vi "Load and Vin SMU Measurement T16.vi"() -> ()   [LabVIEW 2021, in "Dep T16.lvlib"]
doc: "Demonstrates how to use the DC Voltage Output Function to force an output voltage. This example initializes a session, configures the Output Function, Sense, Autorange, Voltage Level and Current Limit, initiates generation, waits for a specified delay, and measures the voltage and current output. This example uses Single Point source mode."
uses:
  Dep T16.lvlib
  controls/Temp T16.ctl
  DMM/DMM T16.lvlib
panel:
  in  "Tektronix Scope":refnum<visa-resource-name>
  out "Division Number":i32
  in  "Sample Rate":dbl=3125000000.0
  in  "Maximum Record Length":dbl=250000000.0 format="%#_6e"
  out "SMU Measurement":dbl format="%.6p"
  in  "SMU DMM":refnum<k15>="Dev1"
  in  "SMU DMM Measurement":T1(ring)
  in  "SMU Resolution in Digits":dbl(ring)=5.5 items=["3 1/2"=3.5, "4 1/2"=4.5, "5 1/2"=5.5, "6 1/2"=6.5, "7 1/2"=7.5]
  out "Load Voltage":dbl caption="SMU Measurement" format="%.6p"
  in  "Load DMM":refnum<k15>="Dev1"
  in  "Load DMM Measurement":T1(ring) caption="SMU DMM Measurement"
  in  "Load SMU":refnum<k15>="Dev1"
  in  "Load SMU Channel":string="0"
  out "Load SMU Current":dbl
  out "Load SMU Voltage":dbl
  in  "error in":errorcluster
  out "error out":errorcluster
  out "Voltage Measurement":dbl caption="Vin SMU Voltage"
  out "Current Measurement":dbl caption="Vin SMU Current"
  in  "Current Limit":dbl=0.01 format="%.3p"
  in  "Voltage Level":dbl=2.0 format="%.5p"
  in  "Vin SMU Channel":string="0"
  in  "Vin SMU":refnum<k15>="Dev1"
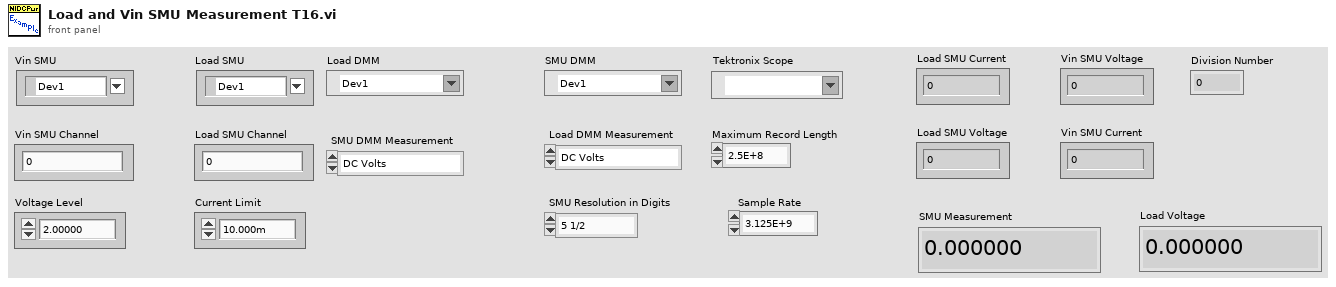
[diagram p1: front panel]
types:
  T1 = enum16{"DC Volts", "AC Volts", "DC Current", "AC Current", "2-wire Resistance", "4-wire Resistance", "Diode", "Frequency", "Period", "AC Volts DC Coupled", "Capacitance", "Inductance", "Temperature"}
  T2 = typedef "Temp T16.ctl" = cluster{"Read?":bool, "Temp":i32}
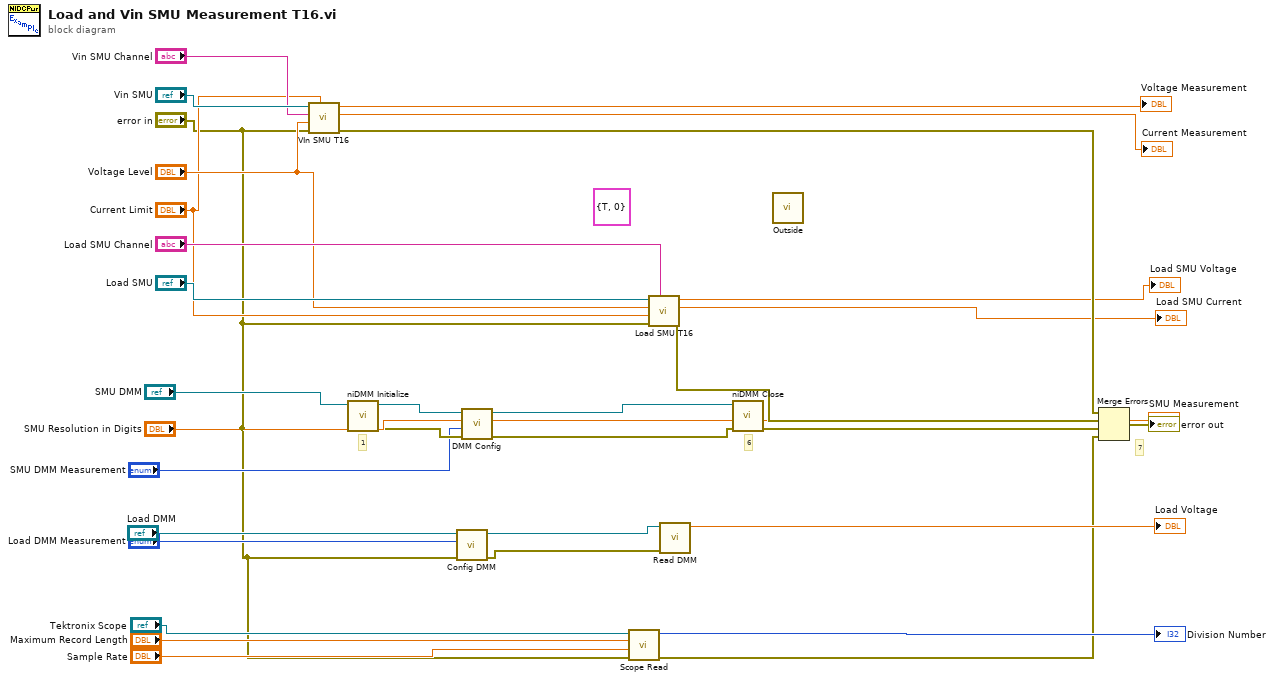
[diagram p0: block diagram]
diagram:
  (unwired) T2 {"Read?"=TRUE, "Temp"=0}
  # "1"
  # "7"
  # "6"
  n1 = call "VIn SMU T16.vi"("Current Limit"="Current Limit", "error in (no error)"="error in", "Voltage Level"="Voltage Level", "Vin SMU Channel"="Vin SMU Channel", "IVI Refnum in"="Vin SMU") -> ("error out"=w32:errorcluster, "Current Measurement"=→"Current Measurement":dbl, "Voltage Measurement"=→"Voltage Measurement":dbl)  [unwired: 4 in]
  n2 = call <instrlib>:"niDMM Initialize.vi"("error in (no error)"="error in", "Instrument Descriptor"="SMU DMM") -> ("error out"=w14:errorcluster, "instrument handle out"=w15:refnum<k15>)  [unwired: 8 in]
  n3 = call "Config DMM.vi"("error in (no error)"="error in", "Load DMM Measurement"="Load DMM Measurement", "IVI Refnum in"="Load DMM") -> ("error out"=w21:errorcluster, "IVI Refnum out"=w20:refnum<k15>)  [unwired: 7 in]
  n4 = call "DMM Config.vi"("error in (no error)"=w14, "SMU DMM Measurement"="SMU DMM Measurement", "SMU Resolution in Digits"="SMU Resolution in Digits", "IVI Refnum in"=w15) -> ("error out"=w3:errorcluster, "Measurement"=→"SMU Measurement":dbl, "IVI Refnum out"=w16:refnum<k15>)  [unwired: 5 in]
  n5 = call "Scope Read.vi"("error in (no error)"="error in", "Sample Rate"="Sample Rate", "Maximum Record Length"="Maximum Record Length", "VISA Refnum in"="Tektronix Scope") -> ("error out"=w4:errorcluster, "Division Number"=→"Division Number":i32)  [unwired: 6 in]
  n6 = call "Load SMU T16.vi"("Load SMU Channel"="Load SMU Channel", "error in (no error)"="error in", "Current Limit"="Current Limit", "Voltage Level"="Voltage Level", "IVI Refnum in"="Load SMU") -> ("error out"=w27:errorcluster, "Numeric"=→"Load SMU Current":dbl, "Numeric 2"=→"Load SMU Voltage":dbl)  [unwired: 4 in]
  n7 = call "Read DMM.vi"("error in (no error)"=w21, "IVI Refnum in"=w20) -> ("Measurement"=→"Load Voltage":dbl)  [unwired: 9 in]
  n8 = call <instrlib>:"niDMM Close.vi"("error in (no error)"=w3, "instrument handle"=w16) -> ("error out"=w10:errorcluster)  [unwired: 9 in]
  n9 = call "Outside.vi"() -> ()  [unwired: 12 in]
  n10 = Merge Errors(w32, w27, w10, w4) -> (→"error out":errorcluster)
